vi "Stitch Image.vi"(8 "Error In":errorcluster, 9 "Manipulator Location":dbl[](array[numeric]), 10 "Process Memory":T1[](array[typedef]), 11 "Source Image":T1) -> (0 "Error Out":errorcluster, 2 "Stitched Image":T1, 3 "Acquired Image":T1)   [LabVIEW 2017]
uses:
  <vilib>/vision/Image Controls.llb/IMAQ Image.ctl
  <vilib>/vision/NI_Vision_Development_Module.lvlib
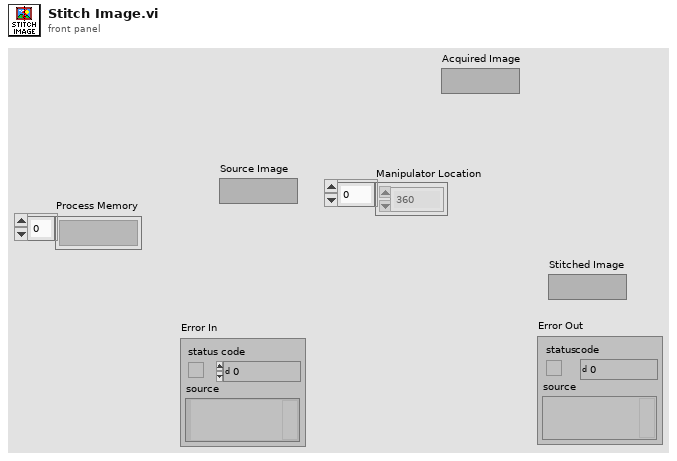
[diagram p1: front panel]
types:
  T1 = typedef "IMAQ Image.ctl" = refnum<image>
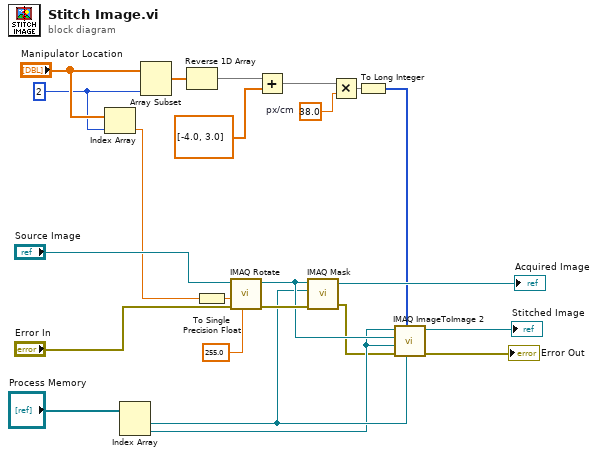
[diagram p0: block diagram]
diagram:
  w4 = 2 ("index")
  w10 = 38.0  # px/cm
  n1 = Index Array(array="Manipulator Location", index=w4) -> (element=w3:dbl)
  n2 = Index Array(array="Process Memory") -> (element #1=w16:T1, element #2=w15:T1)  [unwired: 2 in]
  n3 = Array Subset(array="Manipulator Location", length=w4) -> (w2:dbl[])  [unwired: 1 in]
  n4 = Reverse 1D Array(array=w2) -> (reversed array=w1:dbl[])
  n5 = To Single Precision Float(number=w3) -> (single precision float=w22:sgl)
  n6 = call "IMAQ Rotate"("Replace Value"=sgl 255.0, "error in (no error)"="Error In", "Angle (degrees)"=w22, "Image Src"="Source Image") -> ("error out"=w18:errorcluster, "Image Dst Out"=w17:T1)  [unwired: 6 in]
  n7 = Add(x=w1, y=dbl[] [-4.0, 3.0] ("Array")) -> (x+y=w9:dbl[])
  n8 = call "IMAQ Mask"("error in (no error)"=w18, "Image Mask"=w16, "Image Src"=w17) -> ("error out"=w14:errorcluster, "Image Dst Out"=→"Acquired Image":T1)  [unwired: 2 in]
  n9 = Multiply(x=w9, y=w10) -> (x*y=w6:dbl[])
  n10 = To Long Integer(number=w6) -> (32bit integer=w7:i32[])
  n11 = call "IMAQ ImageToImage 2"("Image Mask"=w16, "Offset Left/Top"=w7, "error in (no error)"=w14, "Image Dst"=w15, "Image Src (Small)"=w17, "Image Src (Large)"=w15) -> ("error out"=→"Error Out":errorcluster, "Image Dst Out"=→"Stitched Image":T1)  [unwired: 4 in]
